vi "Parse Status Header.vi"(7 "Status Header In":string, 11 "error in (no error)":errorcluster) -> (1 "Full Spectrum Starting Wavelength (nm)":dbl, 2 "Full Spectrum Ending Wavelength (nm)":dbl, 3 "Granularity":u32, 6 "Number of Sensors":u16[](array[numeric]), 8 "Status":T2 {"Time Stamp" format="%#_20f"; "Operating Mode" items=["Stand-Alone", "Master", "End Slave", "Middle Slave"]; "Trigger Mode" items=["Untriggered", "Software Triggered", "Hardware Triggered"]; "Full Spectrum Radix" format="%b"}, 10 "Reserved":T1, 15 "error out":errorcluster)   [LabVIEW 2015, in "Micron Optics sm130.lvlib"]
doc: "Parses the status header that is included in every data retrieval."
uses:
  Micron Optics sm130.lvlib
panel:
  out "Errror":u8
  out "error":u8
  out "Array":bool[](array[boolean])
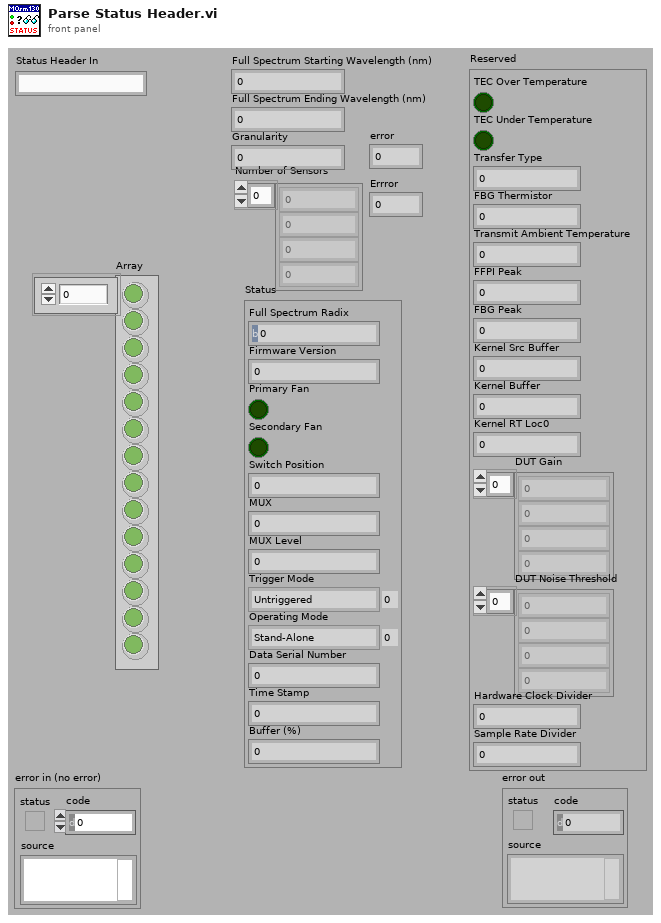
[diagram p1: front panel]
types:
  T1 = cluster{"Transmit Ambient Temperature":dbl, "FBG Thermistor":i16, "FFPI Peak":u16, "FBG Peak":dbl, "Kernel Src Buffer":u16, "Kernel Buffer":u16, "Kernel RT Loc0":u32, "DUT Gain":u16[], "DUT Noise Threshold":u16[], "Hardware Clock Divider":u16, "Sample Rate Divider":u16, "TEC Over Temperature":bool, "TEC Under Temperature":bool, "Transfer Type":u8}
  T2 = cluster{"Full Spectrum Radix":u8, "Firmware Version":u8, "Primary Fan":bool, "Secondary Fan":bool, "Switch Position":u8, "MUX":u8, "Trigger Mode":u8, "Operating Mode":u8, "Data Serial Number":u32, "Time Stamp":dbl, "Buffer (%)":u8, "MUX Level":u8}
  T3 = cluster{"Transmit Ambient Temperature":dbl, "FBG Thermistor":i16, "FFPI Peaks":u16, "FBG Peaks":dbl, "Kernel Src Buffer":u16, "Kernel Buffer":u16, "Kernel RT Loc0":u32, "DUT Gain":u16[], "DUT Noise Threshold":u16[], "Hardware Clock Divider":u16, "Peaks Data Rate Divider":u16, "TEC Over Temperature":bool, "TEC Under Temperature":bool, "Transfer Type":u8}
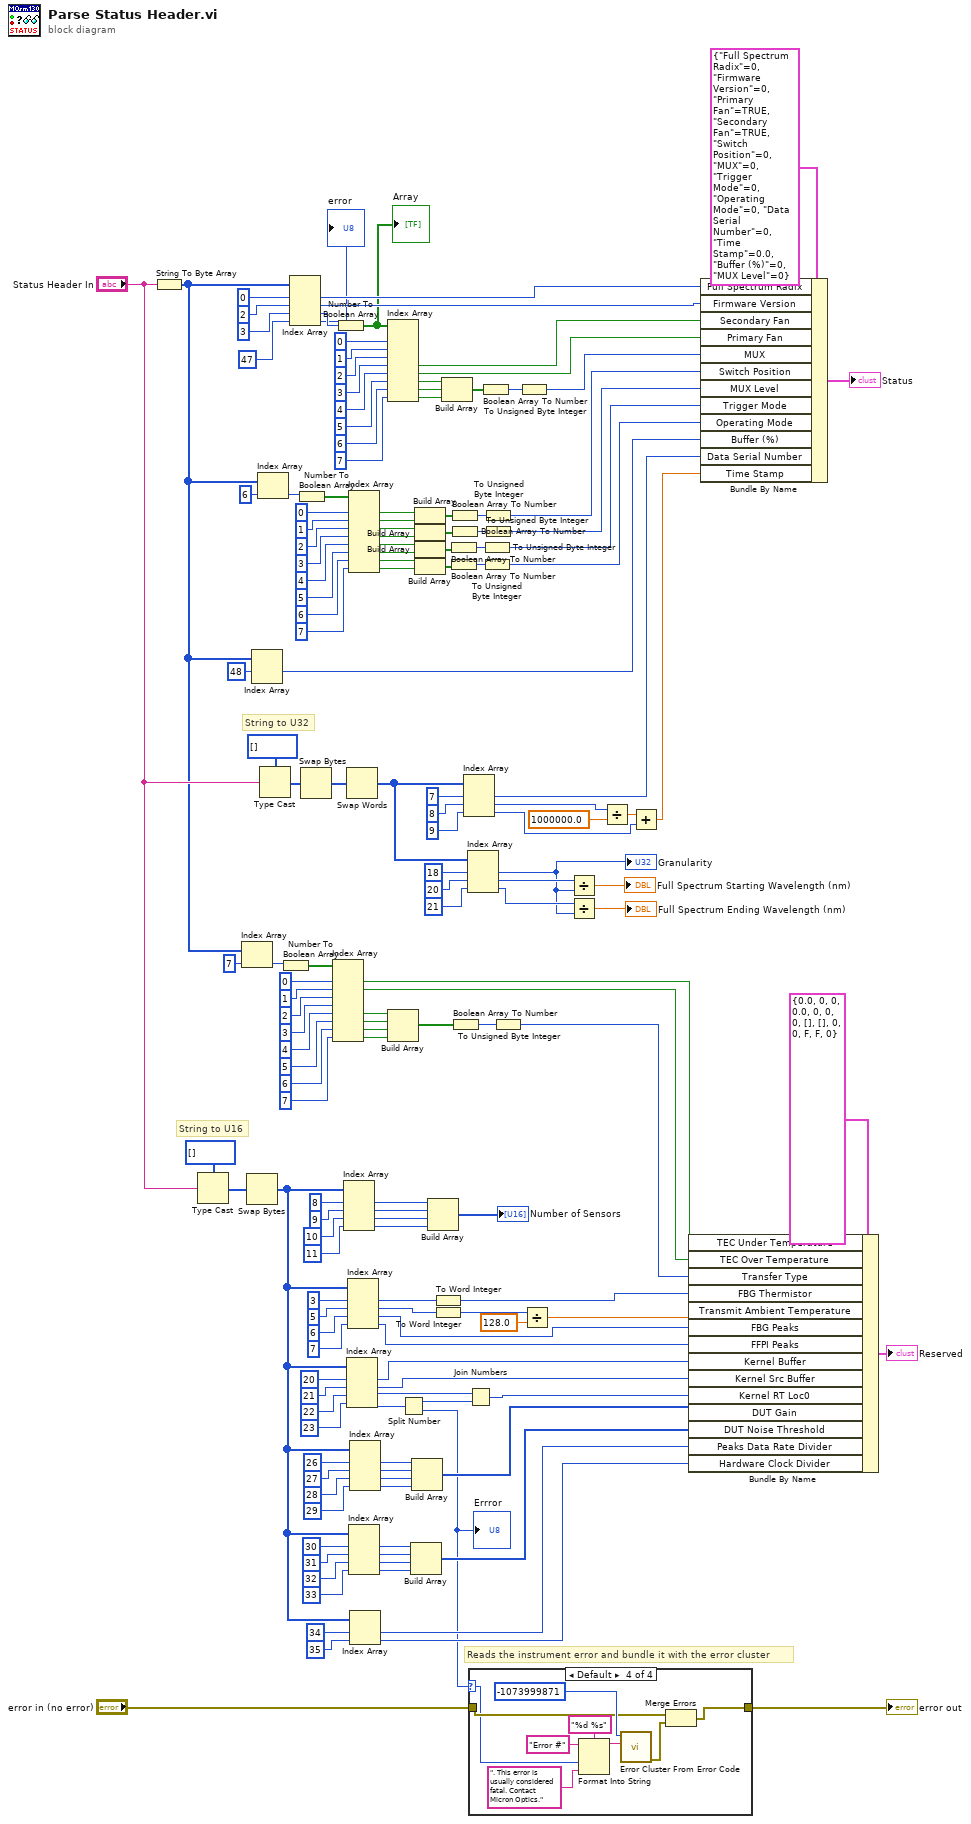
[diagram p0: block diagram]
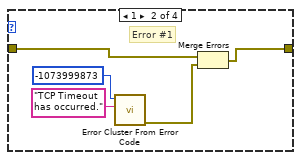
[diagram p3: hidden frame]
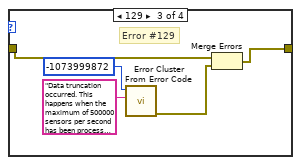
[diagram p4: hidden frame]
diagram:
  # "Reads the instrument error and bundle it with the error cluster"
  # "String to U16"
  # "String to U32"
  n1 = String To Byte Array(string="Status Header In") -> (unsigned byte array=w23:u8[])
  n2 = Type Cast(type=u16[] [], x="Status Header In") -> (*(type *) &x=w113:u16[])
  n3 = Index Array(array=w23, index=7) -> (element=w24:u8)
  n4 = Swap Bytes(anything=w113) -> (byte swapped=w64:u16[])
  n5 = Index Array(array=w23, index #1=48 ("index")) -> (element #1=w58:u8)  [unwired: 1 in, 1 out]
  n6 = Index Array(array=w23, index=6) -> (element=w130:u8)
  n7 = Type Cast(type=u32[] [], x="Status Header In") -> (*(type *) &x=w57:u32[])
  n8 = Number To Boolean Array(number=w24) -> (Boolean array=w33:bool[])
  n9 = Index Array(array=w23, index #1=0 ("index"), index #2=2 ("index"), index #3=3 ("index"), index #4=47 ("index")) -> (element #1=w160:u8, element #2=w159:u8, element #3=w158:u8, element #4=→"error":u8)
  n10 = Number To Boolean Array(number=w130) -> (Boolean array=w139:bool[])
  n11 = Swap Bytes(anything=w57) -> (byte swapped=w55:u32[])
  n12 = Index Array(array=w33, index #1=0 ("index"), index #2=1 ("index"), index #3=2 ("index"), index #4=3 ("index"), index #5=4 ("index"), index #6=5 ("index"), index #7=6 ("index"), index #8=7 ("index")) -> (element #1=w22:bool, element #2=w21:bool, element #5=w20:bool, element #6=w19:bool, element #7=w18:bool, element #8=w17:bool)  [unwired: 2 out]
  n13 = Number To Boolean Array(number=w158) -> (Boolean array=w3:bool[])
  "Array" <- w3
  n14 = Index Array(array=w64, index #1=8 ("index"), index #2=9 ("index"), index #3=10 ("index"), index #4=11 ("index")) -> (element #1=w108:u16, element #2=w107:u16, element #3=w106:u16, element #4=w105:u16)
  n15 = Swap Words(1:w55) -> (0:w41:u32[])
  n16 = Index Array(array=w64, index #1=20 ("index"), index #2=21 ("index"), index #3=22 ("index"), index #4=23 ("index")) -> (element #1=w88:u16, element #2=w87:u16, element #3=w84:u16, element #4=w86:u16)
  n17 = Index Array(array=w64, index #1=3 ("index"), index #2=5 ("index"), index #3=6 ("index"), index #4=7 ("index")) -> (element #1=w103:u16, element #2=w100:u16, element #3=w95:u16, element #4=w93:u16)
  n18 = Index Array(array=w139, index #1=0 ("index"), index #2=1 ("index"), index #3=2 ("index"), index #4=3 ("index"), index #5=4 ("index"), index #6=5 ("index"), index #7=6 ("index"), index #8=7 ("index")) -> (element #1=w129:bool, element #2=w128:bool, element #3=w9:bool, element #4=w8:bool, element #5=w122:bool, element #6=w121:bool, element #7=w118:bool, element #8=w117:bool)
  n19 = Index Array(array=w64, index #1=30 ("index"), index #2=31 ("index"), index #3=32 ("index"), index #4=33 ("index")) -> (element #1=w71:u16, element #2=w70:u16, element #3=w72:u16, element #4=w73:u16)
  n20 = Index Array(array=w64, index #1=26 ("index"), index #2=27 ("index"), index #3=28 ("index"), index #4=29 ("index")) -> (element #1=w77:u16, element #2=w78:u16, element #3=w76:u16, element #4=w75:u16)
  n21 = Index Array(array=w64, index #1=34 ("index"), index #2=35 ("index")) -> (element #1=w61:u16, element #2=w60:u16)
  n22 = Index Array(array=w3, index #1=0 ("index"), index #2=1 ("index"), index #3=2 ("index"), index #4=3 ("index"), index #5=4 ("index"), index #6=5 ("index"), index #7=6 ("index"), index #8=7 ("index")) -> (element #4=w149:bool, element #5=w148:bool, element #6=w146:bool, element #7=w145:bool, element #8=w144:bool)  [unwired: 3 out]
  n23 = Build Array(w20, w19, w18, w17) -> (w16:bool[])
  n24 = Split Number(x=w86) -> (hi(x)=w85:u8, lo(x)=w6:u8)
  "Errror" <- w6
  n25 = Build Array(w71, w70, w72, w73) -> (w65:u16[])
  n26 = Build Array(w77, w78, w76, w75) -> (w74:u16[])
  n27 = Build Array(w129, w128) -> (w126:bool[])
  n28 = Build Array(w9, w8) -> (w11:bool[])
  n29 = Build Array(w122, w121) -> (w124:bool[])
  n30 = Build Array(w118, w117) -> (w119:bool[])
  n31 = Build Array(w108, w107, w106, w105) -> (→"Number of Sensors":u16[])
  n32 = To Word Integer(number=w103) -> (16bit integer=w102:i16)
  n33 = To Word Integer(number=w100) -> (16bit integer=w98:i16)
  n34 = Build Array(w146, w145, w144) -> (w147:bool[])
  n35 = Boolean Array To Number(Boolean array=w124) -> (number=w123:u32)
  n36 = Boolean Array To Number(Boolean array=w119) -> (number=w120:u32)
  n37 = Boolean Array To Number(Boolean array=w126) -> (number=w127:u32)
  n38 = Boolean Array To Number(Boolean array=w11) -> (number=w10:u32)
  n39 = Boolean Array To Number(Boolean array=w16) -> (number=w15:u32)
  n40 = Index Array(array=w41, index #1=7 ("index"), index #2=8 ("index"), index #3=9 ("index")) -> (element #1=w52:u32, element #2=w47:u32, element #3=w46:u32)
  n41 = Join Numbers(hi=w84, lo=w85) -> ((hi.lo)=w83:u32)
  n42 = Index Array(array=w41, index #1=18 ("index"), index #2=20 ("index"), index #3=21 ("index")) -> (element #1=w38:u32, element #2=w40:u32, element #3=w39:u32)
  "Granularity" <- w38
  n43 = case shown="Default" w6 {
    selector: w6 -> [_ _ _ w180]
    tunnel: "error in (no error)" -> [w165 w166 w172 w182]
    tunnel: [w165 w168 w171 w181] -> w4
    frame 0 {
      # "No Error"
    }
    frame 1 {
      # "Error #1"
      n44 = call <vilib>:"Error Cluster From Error Code.vi"("error message (\"\")"="TCP Timeout has occurred." ("error message (\"\")"), "error code (0)"=-1073999873) -> ("error out"=w167:errorcluster)  [unwired: 7 in]
      n45 = Merge Errors(w166, w167) -> (w168:errorcluster)
    }
    frame 129 {
      # "Error #129"
      n46 = call <vilib>:"Error Cluster From Error Code.vi"("error message (\"\")"="Data truncation occurred. This happens when the maximum of 500000 sensors per second has been processed." ("error message (\"\")"), "error code (0)"=-1073999872) -> ("error out"=w173:errorcluster)  [unwired: 7 in]
      n47 = Merge Errors(w172, w173) -> (w171:errorcluster)
    }
    frame Default {
      n48 = Format Into String(format string="%d %s", initial string="Error #", w180, ". This error is usually considered fatal. Contact Micron Optics." ("error message (\"\")")) -> (resulting string=w179:string)  [unwired: 1 in, 1 out]
      n49 = call <vilib>:"Error Cluster From Error Code.vi"("error message (\"\")"=w179, "error code (0)"=-1073999871) -> ("error out"=w183:errorcluster)  [unwired: 7 in]
      n50 = Merge Errors(w182, w183) -> (w181:errorcluster)
    }
  }
  "error out" <- w4
  n51 = Boolean Array To Number(Boolean array=w147) -> (number=w143:u32)
  n52 = To Unsigned Byte Integer(number=w123) -> (unsigned 8bit integer=w13:u8)
  n53 = To Unsigned Byte Integer(number=w120) -> (unsigned 8bit integer=w116:u8)
  n54 = To Unsigned Byte Integer(number=w127) -> (unsigned 8bit integer=w125:u8)
  n55 = To Unsigned Byte Integer(number=w10) -> (unsigned 8bit integer=w7:u8)
  n56 = To Unsigned Byte Integer(number=w15) -> (unsigned 8bit integer=w14:u8)
  n57 = To Unsigned Byte Integer(number=w143) -> (unsigned 8bit integer=w142:u8)
  n58 = Divide(x=w98, y=128.0) -> (x/y=w97:dbl)
  n59 = Divide(x=w40, y=w38) -> (x/y=→"Full Spectrum Starting Wavelength (nm)":dbl)
  n60 = Divide(x=w39, y=w38) -> (x/y=→"Full Spectrum Ending Wavelength (nm)":dbl)
  n61 = Divide(x=w47, y=1000000.0) -> (x/y=w48:dbl)
  n62 = Add(x=w48, y=w46) -> (x+y=w45:dbl)
  n63 = Bundle By Name(cluster=T3 {"Transmit Ambient Temperature"=0.0, "FBG Thermistor"=0, "FFPI Peaks"=0, "FBG Peaks"=0.0, "Kernel Src Buffer"=0, "Kernel Buffer"=0, "Kernel RT Loc0"=0, "DUT Gain"=[], "DUT Noise Threshold"=[], "Hardware Clock Divider"=0, "Peaks Data Rate Divider"=0, "TEC Over Temperature"=FALSE, "TEC Under Temperature"=FALSE, "Transfer Type"=0} ("Reserved 2"), "TEC Under Temperature"=w22, "TEC Over Temperature"=w21, "Transfer Type"=w14, "FBG Thermistor"=w102, "Transmit Ambient Temperature"=w97, "FBG Peaks"=w95, "FFPI Peaks"=w93, "Kernel Buffer"=w88, "Kernel Src Buffer"=w87, "Kernel RT Loc0"=w83, "DUT Gain"=w74, "DUT Noise Threshold"=w65, "Peaks Data Rate Divider"=w61, "Hardware Clock Divider"=w60) -> (→"Reserved":T3)
  n64 = Bundle By Name(cluster=T2 {"Full Spectrum Radix"=0, "Firmware Version"=0, "Primary Fan"=TRUE, "Secondary Fan"=TRUE, "Switch Position"=0, "MUX"=0, "Trigger Mode"=0, "Operating Mode"=0, "Data Serial Number"=0, "Time Stamp"=0.0, "Buffer (%)"=0, "MUX Level"=0} ("Status 2"), "Full Spectrum Radix"=w160, "Firmware Version"=w159, "Secondary Fan"=w149, "Primary Fan"=w148, "MUX"=w142, "Switch Position"=w125, "MUX Level"=w7, "Trigger Mode"=w13, "Operating Mode"=w116, "Buffer (%)"=w58, "Data Serial Number"=w52, "Time Stamp"=w45) -> (→"Status":T2)
